vi "Robocopy.vi"(4 "Output summary to LabVIEW (will no longer be able to see progress in CMD prompt)":bool, 6 "Dest. drive root":path=path "G:/", 7 "Source drive root":path=path "Z:/", 8 "Mode of operation":u16(ring) items=["One way mirror, overwrite destination files even if newer", "One way mirror, don't overwrite newer files at destination", "Two way copy, newest files at both locations"]) -> (0 "Errors out":errorcluster[](array[cluster]), 1 "Commands":string[](array[string]), 3 "End summary":string[](array[string]))   [LabVIEW 2018]
panel:
  # "PN 10/12/2014, \n       16/12/2015"
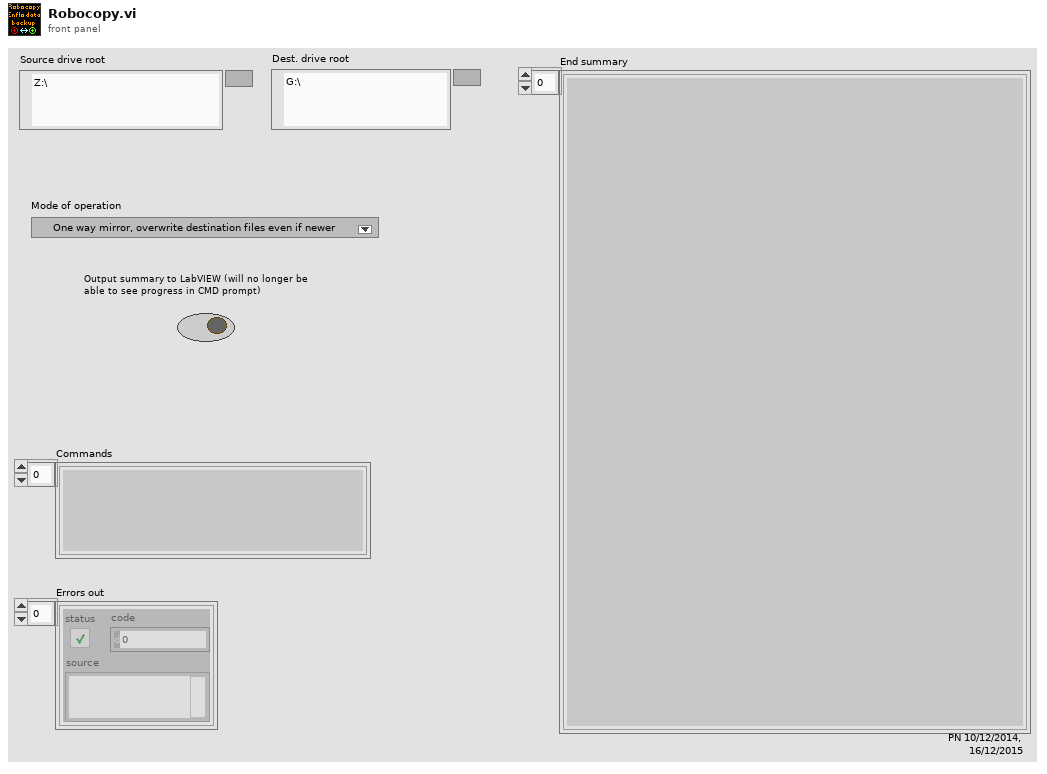
[diagram p1: front panel]
types:
  T1 = enum16{"Zero or one", "One", "Zero or more", "One or more"}
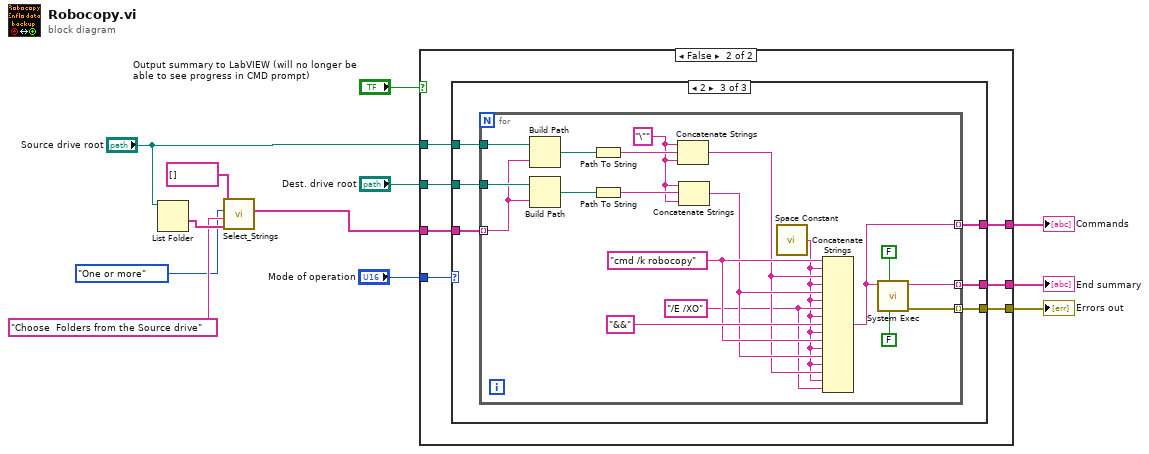
[diagram p0: block diagram]
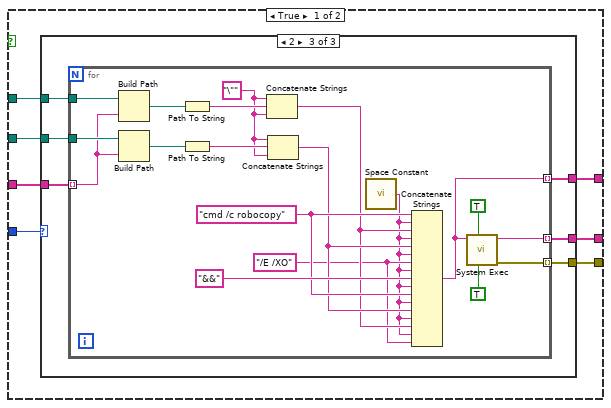
[diagram p2: hidden frame]
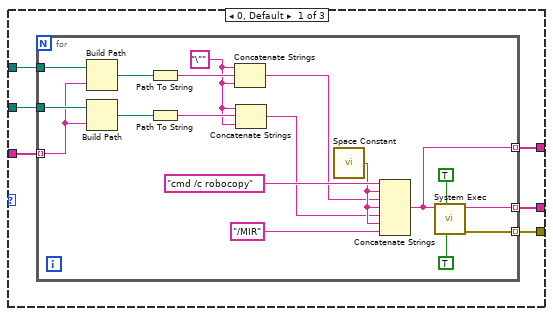
[diagram p3: hidden frame]
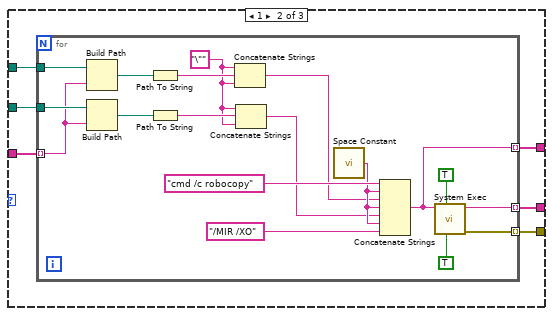
[diagram p4: hidden frame]
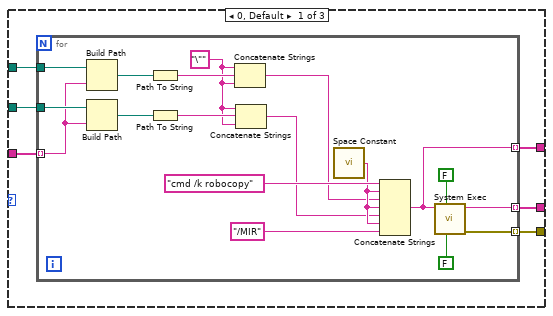
[diagram p5: hidden frame]
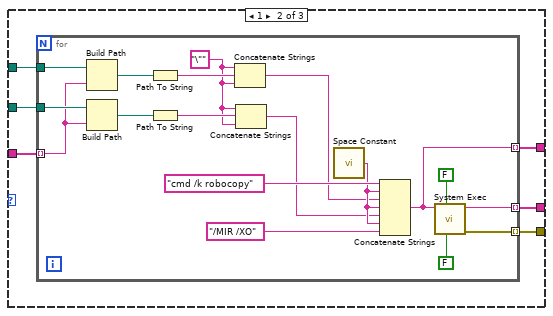
[diagram p6: hidden frame]
diagram:
  n1 = List Folder(path="Source drive root") -> (folder names=w5:string[])  [unwired: 3 in, 3 out]
  n2 = call "Select_Strings.vi"("Available Ch names"=w5, "Message"="Choose  Folders from the Source drive", "Selector mode"=T1."One or more", "Desired Ch names (in)"=string[] []) -> ("Selected Channel Names"=w4:string[])  [unwired: 2 in, 2 out]
  n3 = case shown="False" "Output summary to LabVIEW (will no longer be able to see progress in CMD prompt)" {
    tunnel: "Source drive root" -> [w19 w99]
    tunnel: "Dest. drive root" -> [w18 w98]
    tunnel: w4 -> [w17 w97]
    tunnel: "Mode of operation" -> [w16 w96]
    tunnel: [w15 w95] -> w10
    tunnel: [w14 w94] -> w9
    tunnel: [w13 w93] -> w8
    frame True {
      n4 = case shown="2" w16 {
        tunnel: w19 -> [w25 w49 w73]
        tunnel: w18 -> [w24 w48 w72]
        tunnel: w17 -> [w23 w47 w71]
        tunnel: [w22 w46 w70] -> w14
        tunnel: [w21 w45 w68] -> w15
        tunnel: [w20 w44 w69] -> w13
        frame 0, Default {
          n5 = for {
            tunnel: w25 -> [w41]
            tunnel: w24 -> [w40]
            tunnel: w23 -> [w39] mode=indexing
            tunnel: [w34] -> w21 mode=indexing
            tunnel: [w27] -> w22 mode=indexing
            tunnel: [w26] -> w20 mode=indexing
            w28 = "\"" ("string")
            n6 = Build Path(base path=w41, name or relative path=w39) -> (appended path=w37:path)
            n7 = Build Path(base path=w40, name or relative path=w39) -> (appended path=w36:path)
            n8 = Path To String(path=w37) -> (string=w32:string)
            n9 = Path To String(path=w36) -> (string=w30:string)
            n10 = Concatenate Strings(w28, w32, w28) -> (w31:string)
            n11 = Concatenate Strings(w28, w30, w28) -> (w29:string)
            n12 = call <vilib>:"Space Constant.vi"() -> ("String"=w33:string)
            n13 = Concatenate Strings("cmd /c robocopy", w33, w31, w33, w29, w33, "/MIR" ("string")) -> (w27:string)
            n14 = call <vilib>:"System Exec.vi"("run minimized? (F)"=TRUE, "wait until completion? (T)"=TRUE, "command line"=w27) -> ("error out"=w34:errorcluster, "standard output"=w26:string)  [unwired: 5 in, 2 out]
          }
        }
        frame 1 {
          n15 = for {
            tunnel: w49 -> [w65]
            tunnel: w48 -> [w64]
            tunnel: w47 -> [w63] mode=indexing
            tunnel: [w58] -> w45 mode=indexing
            tunnel: [w51] -> w46 mode=indexing
            tunnel: [w50] -> w44 mode=indexing
            w52 = "\"" ("string")
            n16 = Build Path(base path=w65, name or relative path=w63) -> (appended path=w61:path)
            n17 = Build Path(base path=w64, name or relative path=w63) -> (appended path=w60:path)
            n18 = Path To String(path=w61) -> (string=w56:string)
            n19 = Path To String(path=w60) -> (string=w54:string)
            n20 = Concatenate Strings(w52, w56, w52) -> (w55:string)
            n21 = Concatenate Strings(w52, w54, w52) -> (w53:string)
            n22 = call <vilib>:"Space Constant.vi"() -> ("String"=w57:string)
            n23 = Concatenate Strings("cmd /c robocopy", w57, w55, w57, w53, w57, "/MIR /XO" ("string")) -> (w51:string)
            n24 = call <vilib>:"System Exec.vi"("run minimized? (F)"=TRUE, "wait until completion? (T)"=TRUE, "command line"=w51) -> ("error out"=w58:errorcluster, "standard output"=w50:string)  [unwired: 5 in, 2 out]
          }
        }
        frame 2 {
          n25 = for {
            tunnel: w73 -> [w90]
            tunnel: w72 -> [w89]
            tunnel: w71 -> [w88] mode=indexing
            tunnel: [w82] -> w70 mode=indexing
            tunnel: [w81] -> w69 mode=indexing
            tunnel: [w75] -> w68 mode=indexing
            w83 = "\"" ("string")
            w76 = "/E /XO" ("string")
            w79 = "cmd /c robocopy"
            n26 = Build Path(base path=w90, name or relative path=w88) -> (appended path=w87:path)
            n27 = Build Path(base path=w89, name or relative path=w88) -> (appended path=w86:path)
            n28 = Path To String(path=w87) -> (string=w85:string)
            n29 = Path To String(path=w86) -> (string=w84:string)
            n30 = Concatenate Strings(w83, w85, w83) -> (w77:string)
            n31 = Concatenate Strings(w83, w84, w83) -> (w78:string)
            n32 = call <vilib>:"Space Constant.vi"() -> ("String"=w74:string)
            n33 = Concatenate Strings(w79, w74, w77, w74, w78, w74, w76, w74, "&&" ("string"), w74, w79, w74, w78, w74, w77, w74, w76) -> (w82:string)
            n34 = call <vilib>:"System Exec.vi"("run minimized? (F)"=TRUE, "wait until completion? (T)"=TRUE, "command line"=w82) -> ("error out"=w75:errorcluster, "standard output"=w81:string)  [unwired: 5 in, 2 out]
          }
        }
      }
    }
    frame False {
      n35 = case shown="2" w96 {
        tunnel: w99 -> [w105 w129 w153]
        tunnel: w98 -> [w104 w128 w152]
        tunnel: w97 -> [w103 w127 w151]
        tunnel: [w102 w126 w150] -> w94
        tunnel: [w101 w125 w148] -> w95
        tunnel: [w100 w124 w149] -> w93
        frame 0, Default {
          n36 = for {
            tunnel: w105 -> [w121]
            tunnel: w104 -> [w120]
            tunnel: w103 -> [w119] mode=indexing
            tunnel: [w114] -> w101 mode=indexing
            tunnel: [w107] -> w102 mode=indexing
            tunnel: [w106] -> w100 mode=indexing
            w108 = "\"" ("string")
            n37 = Build Path(base path=w121, name or relative path=w119) -> (appended path=w117:path)
            n38 = Build Path(base path=w120, name or relative path=w119) -> (appended path=w116:path)
            n39 = Path To String(path=w117) -> (string=w112:string)
            n40 = Path To String(path=w116) -> (string=w110:string)
            n41 = Concatenate Strings(w108, w112, w108) -> (w111:string)
            n42 = Concatenate Strings(w108, w110, w108) -> (w109:string)
            n43 = call <vilib>:"Space Constant.vi"() -> ("String"=w113:string)
            n44 = Concatenate Strings("cmd /k robocopy", w113, w111, w113, w109, w113, "/MIR" ("string")) -> (w107:string)
            n45 = call <vilib>:"System Exec.vi"("run minimized? (F)"=FALSE, "wait until completion? (T)"=FALSE, "command line"=w107) -> ("error out"=w114:errorcluster, "standard output"=w106:string)  [unwired: 5 in, 2 out]
          }
        }
        frame 1 {
          n46 = for {
            tunnel: w129 -> [w145]
            tunnel: w128 -> [w144]
            tunnel: w127 -> [w143] mode=indexing
            tunnel: [w138] -> w125 mode=indexing
            tunnel: [w131] -> w126 mode=indexing
            tunnel: [w130] -> w124 mode=indexing
            w132 = "\"" ("string")
            n47 = Build Path(base path=w145, name or relative path=w143) -> (appended path=w141:path)
            n48 = Build Path(base path=w144, name or relative path=w143) -> (appended path=w140:path)
            n49 = Path To String(path=w141) -> (string=w136:string)
            n50 = Path To String(path=w140) -> (string=w134:string)
            n51 = Concatenate Strings(w132, w136, w132) -> (w135:string)
            n52 = Concatenate Strings(w132, w134, w132) -> (w133:string)
            n53 = call <vilib>:"Space Constant.vi"() -> ("String"=w137:string)
            n54 = Concatenate Strings("cmd /k robocopy", w137, w135, w137, w133, w137, "/MIR /XO" ("string")) -> (w131:string)
            n55 = call <vilib>:"System Exec.vi"("run minimized? (F)"=FALSE, "wait until completion? (T)"=FALSE, "command line"=w131) -> ("error out"=w138:errorcluster, "standard output"=w130:string)  [unwired: 5 in, 2 out]
          }
        }
        frame 2 {
          n56 = for {
            tunnel: w153 -> [w170]
            tunnel: w152 -> [w169]
            tunnel: w151 -> [w168] mode=indexing
            tunnel: [w162] -> w150 mode=indexing
            tunnel: [w161] -> w149 mode=indexing
            tunnel: [w155] -> w148 mode=indexing
            w163 = "\"" ("string")
            w156 = "/E /XO" ("string")
            w159 = "cmd /k robocopy"
            n57 = Build Path(base path=w170, name or relative path=w168) -> (appended path=w167:path)
            n58 = Build Path(base path=w169, name or relative path=w168) -> (appended path=w166:path)
            n59 = Path To String(path=w167) -> (string=w165:string)
            n60 = Path To String(path=w166) -> (string=w164:string)
            n61 = Concatenate Strings(w163, w165, w163) -> (w157:string)
            n62 = Concatenate Strings(w163, w164, w163) -> (w158:string)
            n63 = call <vilib>:"Space Constant.vi"() -> ("String"=w154:string)
            n64 = Concatenate Strings(w159, w154, w157, w154, w158, w154, w156, w154, "&&" ("string"), w154, w159, w154, w158, w154, w157, w154, w156) -> (w162:string)
            n65 = call <vilib>:"System Exec.vi"("run minimized? (F)"=FALSE, "wait until completion? (T)"=FALSE, "command line"=w162) -> ("error out"=w155:errorcluster, "standard output"=w161:string)  [unwired: 5 in, 2 out]
          }
        }
      }
    }
  }
  "Errors out" <- w10
  "Commands" <- w9
  "End summary" <- w8
